vi "modcorrection.vi"(2 "frequency (T)":dbl[](array[numeric]) format="%.2f", 3 "mod depth (mT)":dbl=60.0 format="%.2f", 4 "field (T)":dbl=10.0 format="%.2f") -> (0 "J (n)":dbl[](array[numeric]) format="%.2f", 1 "lambda":dbl[](array[numeric]) format="%.2f")   [LabVIEW 2018]
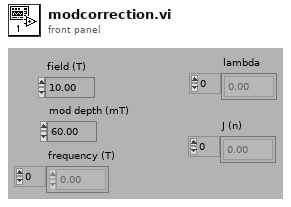
[diagram p1: front panel]
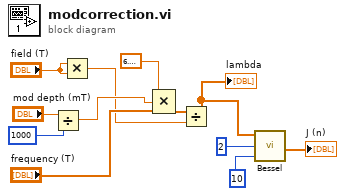
[diagram p0: block diagram]
diagram:
  n1 = Divide(x="mod depth (mT)", y=1000) -> (x/y=w9:dbl)
  n2 = Multiply(x="field (T)", y="field (T)") -> (x*y=w5:dbl)
  n3 = Compound Arithmetic op=MULTIPLY(6.283185307179586, w9, "frequency (T)") -> (w6:dbl[])
  n4 = Divide(x=w6, y=w5) -> (x/y=w4:dbl[])
  "lambda" <- w4
  n5 = call "Bessel.vi"("# terms"=10, "order"=2, "lambda"=w4) -> ("B (lambda"=→"J (n)":dbl[])
